vi "String to TimerPGM.vi"(8 "error in":errorcluster, 9 "Step String":string, 10 "PGM String":string, 11 "Op./Stop Mode":T1) -> (0 "error out":errorcluster, 1 "Step No.":i32, 2 "PGM No.":i32, 3 "Op./Stop Mode Out":T1)   [LabVIEW 2016, in "Environment Chamber.lvlib" / "Climatic Chamber.lvlib"]
uses:
  Climatic Chamber.lvlib
  Type Defs/Operation_Stop Mode Enum.ctl
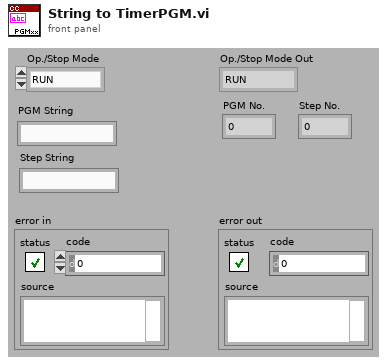
[diagram p1: front panel]
types:
  T1 = typedef "Environment Chamber.lvlib/Climatic Chamber.lvlib/Operation_Stop Mode Enum.ctl" = enum16{"RUN", "CONSTANT", "STANDBY", "OFF"}
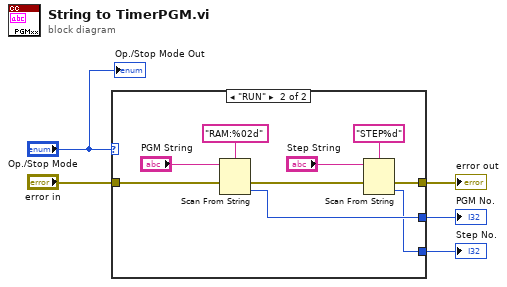
[diagram p0: block diagram]
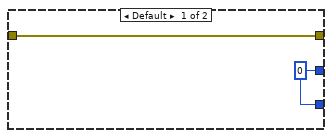
[diagram p2: hidden frame]
diagram:
  n1 = case shown="\"RUN\"" "Op./Stop Mode" {
    tunnel: "error in" -> [w7 w13]
    tunnel: [w7 w11] -> w4
    tunnel: [w6 w9] -> w2
    tunnel: [w6 w8] -> w1
    frame Default {
      w6 = 0
    }
    frame "RUN" {
      n2 = Scan From String(format string="RAM:%02d", input string="PGM String", error in=w13) -> (error out=w12:errorcluster, output 1=w9:i32)  [unwired: 2 in, 2 out]
      n3 = Scan From String(format string="STEP%d", input string="Step String", error in=w12) -> (error out=w11:errorcluster, output 1=w8:i32)  [unwired: 2 in, 2 out]
    }
  }
  "error out" <- w4
  "PGM No." <- w2
  "Step No." <- w1
  "Op./Stop Mode Out" <- "Op./Stop Mode"
